vi "试件吸声量AT计算.vi"(1 "混响室吸声量A1":dbl[](array[numeric]), 2 "混响室吸声量A2":dbl[](array[numeric])) -> (7 "试件吸声量AT":dbl[](array[numeric]))   [LabVIEW 2020]
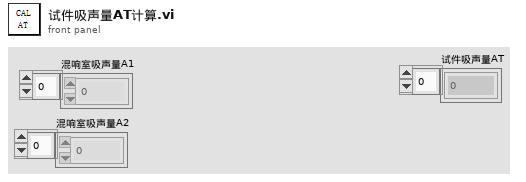
[diagram p1: front panel]
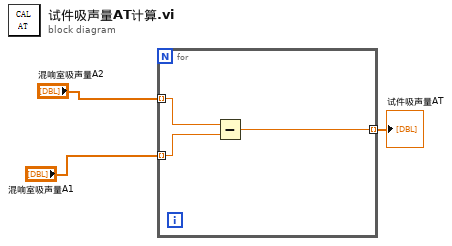
[diagram p0: block diagram]
diagram:
  n1 = for {
    tunnel: "混响室吸声量A2" -> [w6] mode=indexing
    tunnel: "混响室吸声量A1" -> [w5] mode=indexing
    tunnel: [w4] -> w3 mode=indexing
    n2 = Subtract(x=w6, y=w5) -> (x-y=w4:dbl)
  }
  "试件吸声量AT" <- w3
